vi "Vision Processing.vi"(4 "error in (no error)":errorcluster, 6 "CameraDevRef":T1) -> ()   [LabVIEW 2011]
uses:
  <vilib>/Rock Robotics/WPI/Camera/WPI_CameraDevRef.ctl
  Robot Global Data.vi
  <vilib>/vision/NI_Vision_Development_Module.lvlib
panel:
  in  "Default Shooter Speed Dump":dbl=0.42
  in  "Default Shooter Speed Shoot":dbl=0.705
  in  "Scale":dbl=0.85
  in  "Minimum Power":dbl=0.22
  out "Aspect Ratio":dbl[](array[numeric])
  out "Offset":dbl
  in  "Max Distance for 1 hoop":dbl=8.0
  out "Raw Turret":dbl
  in  "Run Calculations":bool=TRUE
  out "Target X Coord":dbl
  out "Target Distance":dbl
  out "Target Y Coord":dbl
  out "Distance Array":dbl[](array[numeric])
  in  "Dead Band":dbl=0.09
  out "Number of Rectangles Visible":dbl
  out "Y Position Array":dbl[](array[numeric])
  out "X Position Array":dbl[](array[numeric])
  in  "View":bool
  out "Target Info":T2(array[cluster])
  in  "Area Size Limit":i32=444
  in  "Particle Count Limit":i32=8
  in  "Score Limits":T3={"Rect Coverage"=76.0, "Aspect Ratio"=40.0, "X Edge Strength"=40.0, "Y Edge Strength"=60.0}
  in  "Processing":enum32{"Color", "Intensity", "Intensity Open"}(tab)=enum."Intensity"
  in  "Luminance":i32=255
  in  "Saturation":i32=255
  in  "Hue":i32(knob)=65 scale=0.0..255.0
  in  "Margins":cluster{"Hue":i32, "Sat":i32, "Lum":i32}={"Hue"=20, "Sat"=27, "Lum"=30} {"Sat" scale=0.0..40.0; "Lum" scale=0.0..40.0; "Hue" scale=0.0..40.0}
  in  "Range":cluster{"Lower value":sgl, "Upper value":sgl}={"Lower value"=151.52174, "Upper value"=255.0} {"Lower value" scale=0.0..255.0; "Upper value" scale=0.0..255.0}
  in  "Range":cluster{"Lower value":sgl, "Upper value":sgl}={"Lower value"=123.804344, "Upper value"=255.0} {"Lower value" scale=0.0..255.0; "Upper value" scale=0.0..255.0}
  in  "View":bool
  out "Processed Image":T4(plugin-control)
  out "Original Image":T4(plugin-control)
  # "Instructions:\nProcessing the reflective tape that is illuminated by a ring light can be based\non color or light intensity.\nParticles within the image are scored by rectangle coverage, aspect ratio, and\nfor being hollow with a bold edge. A particle is considered a target if all scores\nare above the score limits. Particles can be annotated -- surrounded by\na rectangle and scores drawn to the left .\nTo control the number of particles being scored, use the count limit and the size\nlimit."
  # "(in)"
  # "To debug, Enable using the View button.\nFor color processing, you can click in the image to select the color for processing."
  # "Enable by clicking the View button.\nGreen scores are above the limit, orange are below. Inner/outer rect\nindicates all passed."
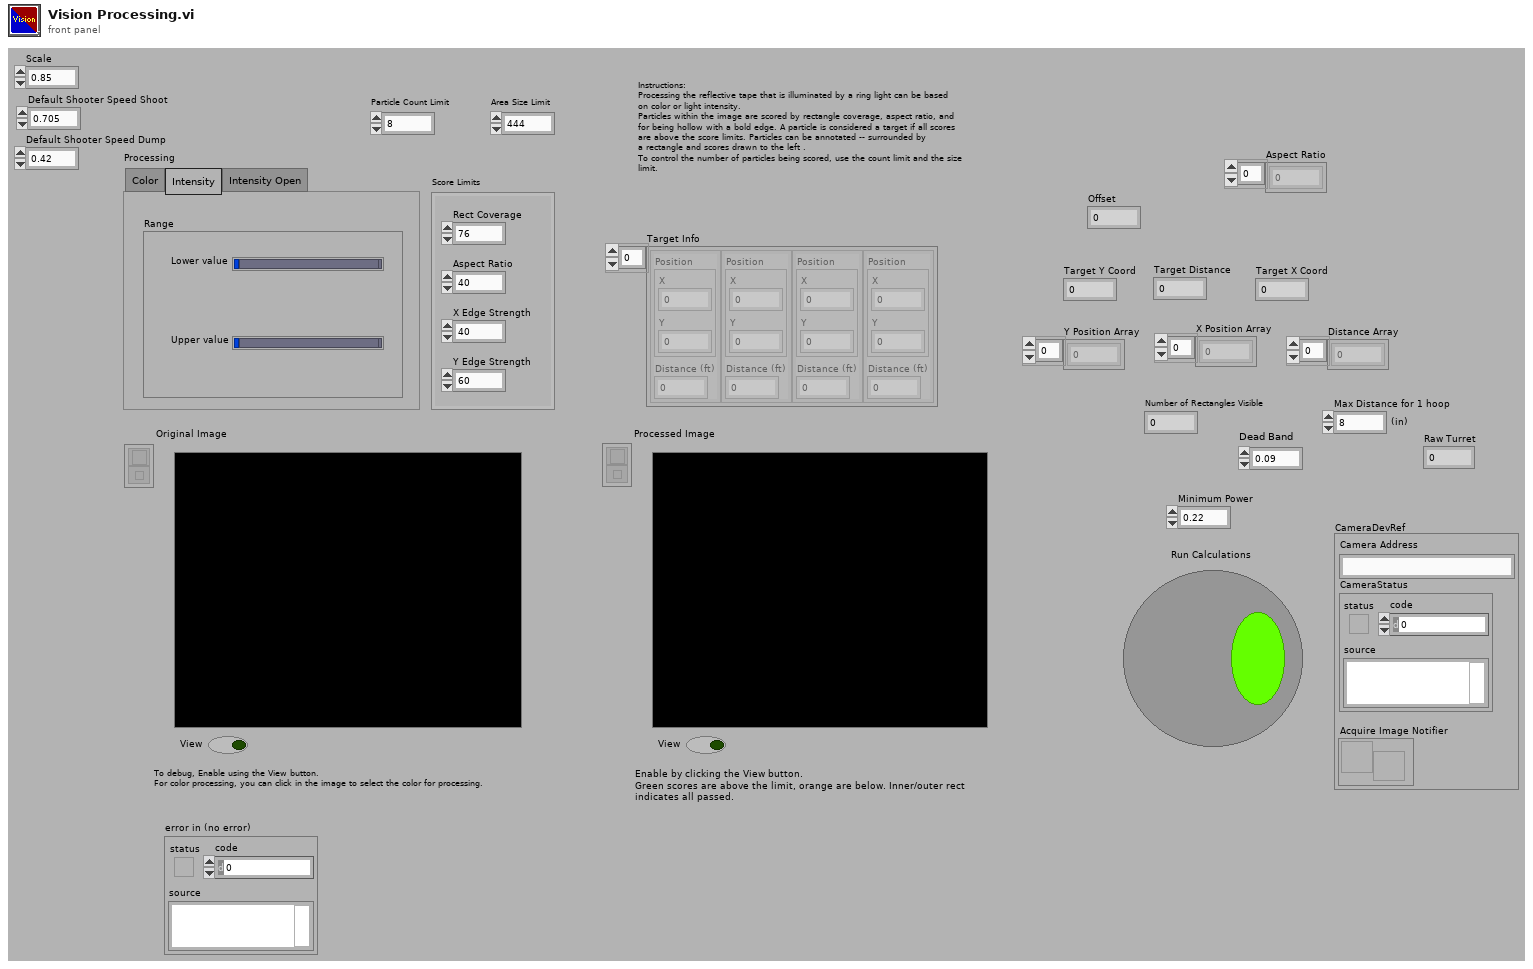
[diagram p1: front panel]
types:
  T1 = typedef "WPI_CameraDevRef.ctl" = cluster{"Camera Address":string, "CameraStatus":errorcluster, "Acquire Image Notifier":refnum<notifier>}
  T2 = cluster{"Position":cluster{"X":dbl, "Y":dbl}, "Distance (ft)":dbl}[]
  T3 = cluster{"Rect Coverage":dbl, "Aspect Ratio":dbl, "X Edge Strength":dbl, "Y Edge Strength":dbl}
  T4 = typedef "IMAQ Image.ctl" = refnum<image>
  T5 = typedef "Image Type" = u32
  T6 = enum32{"AutoM", "Close", "Dilate", "Erode", "Gradient", "Gradient out", "Gradient in", "Hit miss", "Open", "PClose", "POpen", "Thick", "Thin"}
  T7 = typedef "WPI_CameraImageSize.ctl" = enum16{"640x480", "320x240", "160x120"}
  T8 = cluster{"fps":i32, "compression":i32, "Image Size":T7}
  T9 = cluster{cluster{"Left":dbl, "Top":dbl, "Right":dbl, "Bottom":dbl}, dbl[]}[]
  T10 = cluster{"Left":dbl, "Top":dbl, "Right":dbl, "Bottom":dbl}
  T11 = cluster{"Target Center (-1 to 1)":cluster{"X":dbl, "Y":dbl}, "Distance (ft)":dbl}
  T12 = cluster{"Target Center (-1 to 1)":cluster{"X":dbl, "Y":dbl}, "Distance (ft)":dbl}[]
  T13 = typedef "WPI_JoystickDevRef.ctl" = cluster{"Device":T14}
  T14 = typedef "WPI_JoystickDeviceEnum.ctl" = enum16{"USB 1", "USB 2", "USB 3", "USB 4", "Kinect 1", "Kinect 2"}
  T15 = typedef "WPI_JoystickButtonState.ctl" = cluster{"Button 1":bool, "Button 2":bool, "Button 3":bool, "Button 4":bool, "Button 5":bool, "Button 6":bool, "Button 7":bool, "Button 8":bool, "Button 9":bool, "Button 10":bool, "Button 11":bool, "Button 12":bool}
  T16 = cluster{"axis 1 (x)":dbl, "axis 2 (y)":dbl, "axis 3 (throttle)":dbl, "axis 4":dbl, "axis 5":dbl, "axis 6":dbl}
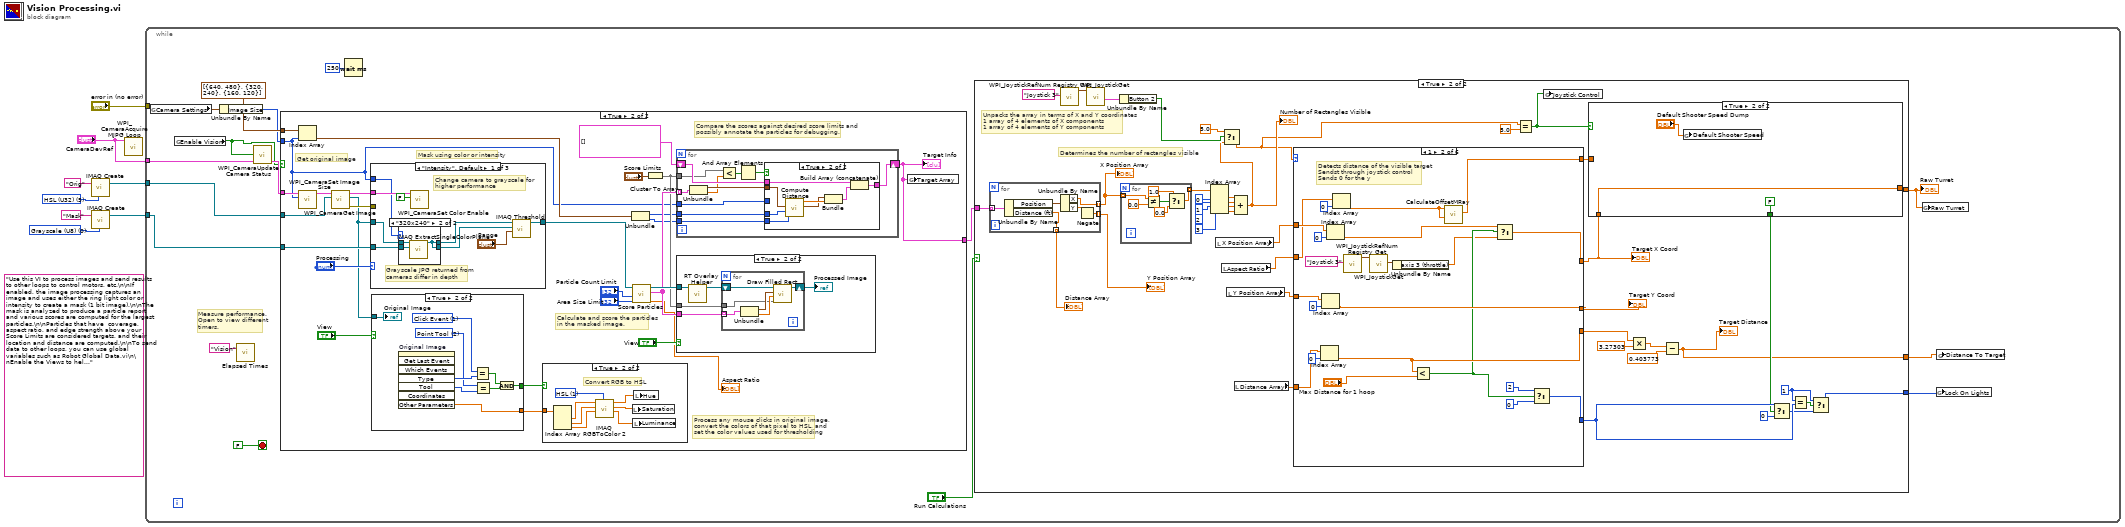
[diagram p0: block diagram]
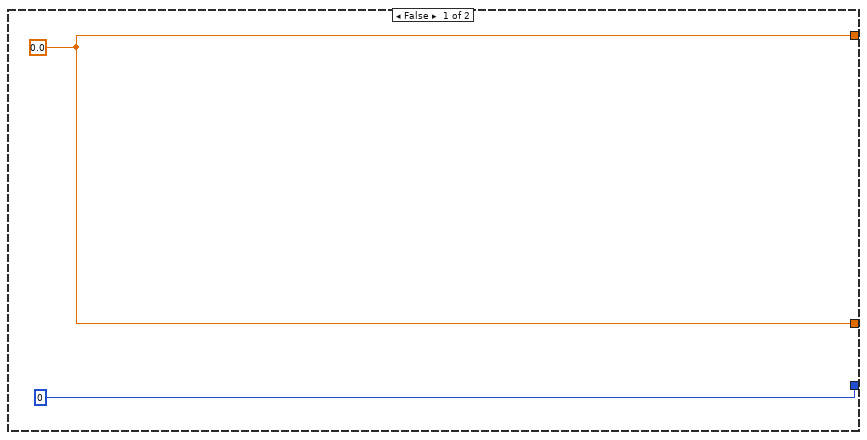
[diagram p2: hidden frame]
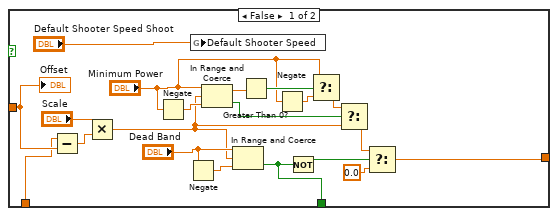
[diagram p3: hidden frame]
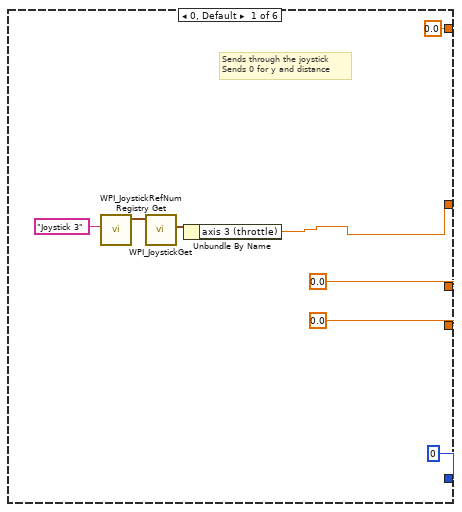
[diagram p4: hidden frame]
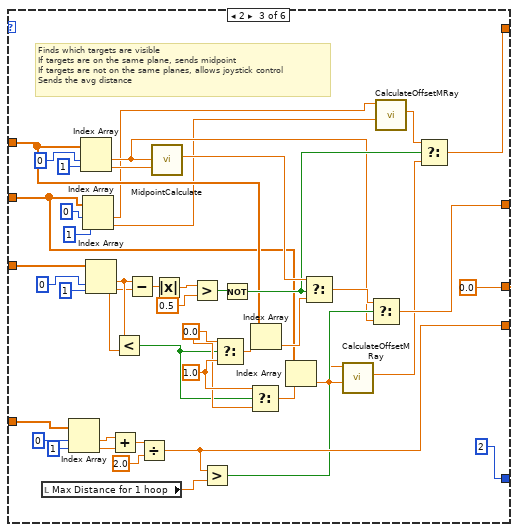
[diagram p5: hidden frame]
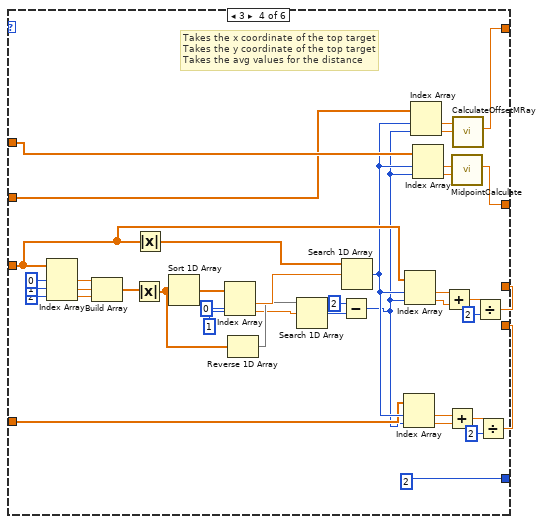
[diagram p6: hidden frame]
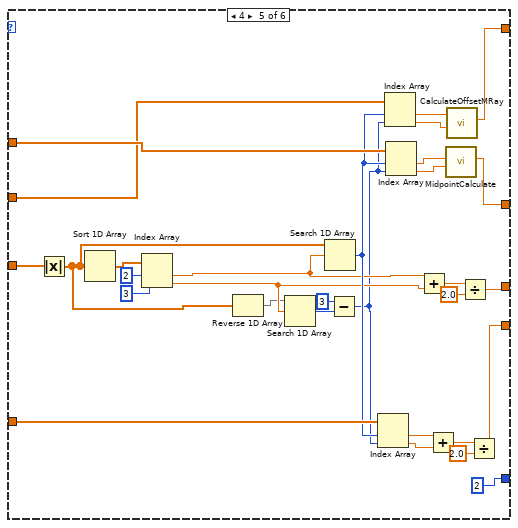
[diagram p7: hidden frame]
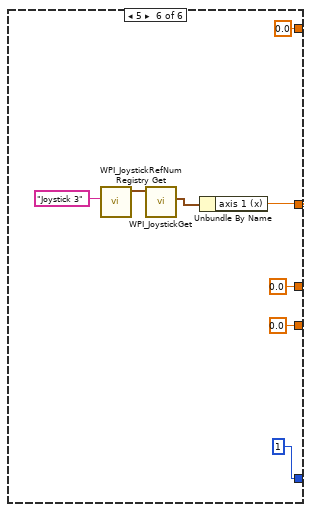
[diagram p8: hidden frame]
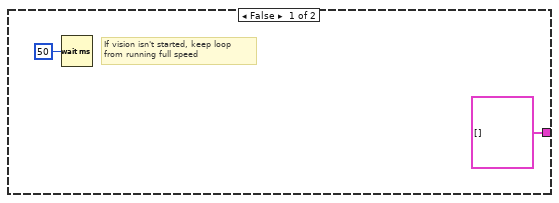
[diagram p9: hidden frame]
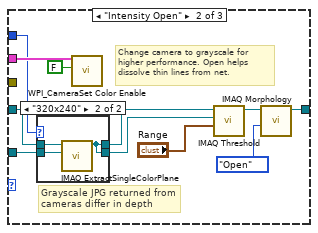
[diagram p12: hidden frame]
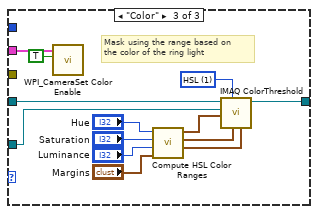
[diagram p14: hidden frame]
diagram:
  w3 = T5 0 items=["Grayscale (U8)", "Grayscale (I16)", "Grayscale (SGL)", "Complex (CSG)", "RGB (U32)", "HSL (U32)", "RGB (U64)", "Grayscale (U16)"] ("Image Type")
  (unwired) "Use this VI to process images and send results to other loops to control motors, etc.\n\nIf enabled, the image processing captures an image and uses either the ring light color or intensity to create a mask (1 bit image).\n\nThe mask is analyzed to produce a particle report and various scores are computed for the largest particles.\n\nParticles that have  coverage, aspect ratio, and edge strength above your Score Limits are considered targets, and their location and distance are computed.\n\nTo send data to other loops, you can use global variables such as Robot Global Data.vi\n\nEnable the Views to help debug color settings. Disable the View to speed up processing."
  w7 = T5 5 items=["Grayscale (U8)", "Grayscale (I16)", "Grayscale (SGL)", "Complex (CSG)", "RGB (U32)", "HSL (U32)", "RGB (U64)", "Grayscale (U16)"] ("Image Type")
  n1 = call "IMAQ Create"("Image Name"="Orig", "Image Type"=w7) -> ("New Image"=w6:T4)  [unwired: 2 in, 2 out]
  n2 = call "IMAQ Create"("Image Name"="Mask", "Image Type"=w3) -> ("New Image"=w1:T4)  [unwired: 2 in, 2 out]
  n3 = call <vilib>:"WPI_CameraAcquire MJPG Loop.vi"("CameraDevRef"="CameraDevRef") -> ()  [unwired: 11 in]
  n4 = while {
    tunnel: w6 -> [w23]
    tunnel: "CameraDevRef" -> [w22]
    tunnel: "error in (no error)" -> [_]
    tunnel: w1 -> [w18]
    stop <- FALSE stop-if-true
    # "Measure performance.\nOpen to view different\ntimers."
    n5 = global read "Robot Global Data.vi" "Camera Settings"() -> (w16:T8)
    n6 = global read "Robot Global Data.vi" "Enable Vision"() -> (w20:bool)
    n7 = Unbundle By Name(w16) -> ("Image Size"=w15:T7)
    n8 = call "Elapsed Times.vi"("Call Name"="Vision") -> ()  [unwired: 2 in, 1 out]
    n9 = call <vilib>:"WPI_CameraUpdate Camera Status.vi"("CameraDevRef In"=w22, "Enable Vision"=w20) -> ("CameraDevRef Out"=w21:T1)  [unwired: 3 in]
    n10 = case shown="True" w20 {
      tunnel: w23 -> [_ w277]
      tunnel: w21 -> [_ w273]
      tunnel: w18 -> [_ w264]
      tunnel: cluster{i32, i32}[] [{640, 480}, {320, 240}, {160, 120}] -> [_ w268]
      tunnel: w15 -> [_ w261]
      tunnel: [T2 [] w262] -> w14
      frame False {
        # "If vision isn't started, keep loop\nfrom running full speed"
        n11 = Wait (ms)(milliseconds to wait=u32 50) -> ()  [unwired: 1 out]
      }
      frame True {
        # "Compare the scores against desired score limits and\npossibly annotate the particles for debugging."
        # "Process any mouse clicks in original image,\nconvert the colors of that pixel to HSL, and\nset the color values used for thresholding"
        # "Calculate and score the particles\nin the masked image."
        # "Mask using color or intensity"
        # "Get original image"
        n12 = call <vilib>:"WPI_CameraSet Image Size.vi"("Image Size"=w261, "CameraDevRef"=w273) -> ("CameraDevRef Out"=w274:T1)  [unwired: 8 in, 1 out]
        n13 = Index Array(array=w268, index=w261) -> (element=w265:cluster{i32, i32})
        n14 = call <vilib>:"WPI_CameraGet Image.vi"("Image"=w277, "CameraDevRef"=w274) -> ("error out"=w275:errorcluster, "Image Out"=w263:T4, "CameraDevRef Out"=w276:T1)  [unwired: 7 in]
        n15 = case shown="\"Intensity\", Default" "Processing" {
          tunnel: w263 -> [w299 w311 w337]
          tunnel: [w302 w316 w336] -> w271
          tunnel: w276 -> [w300 w314 w327]
          tunnel: w275 -> [_ _ _]
          tunnel: w264 -> [w298 w312 w325]
          tunnel: w261 -> [w297 w313 _]
          frame "Intensity", Default {
            # "Grayscale JPG returned from\ncameras differ in depth"
            # "Change camera to grayscale for\nhigher performance"
            n16 = case shown="\"320x240\"" w297 {
              tunnel: w299 -> [w305 w308]
              tunnel: w298 -> [w304 w307]
              tunnel: [w305 w306] -> w296
              tunnel: [w304 w306] -> w295
              frame "640x480", Default {
              }
              frame "320x240" {
                n17 = call "IMAQ ExtractSingleColorPlane"("Image Dst"=w307, "Image Src"=w308) -> ("Image Dst Out"=w306:T4)  [unwired: 8 in, 1 out]
              }
            }
            n18 = call <vilib>:"WPI_CameraSet Color Enable.vi"("Color Enabled"=FALSE, "CameraDevRef"=w300) -> ()  [unwired: 8 in, 2 out]
            n19 = call "IMAQ Threshold"("Range"="Range", "Image Dst"=w295, "Image Src"=w296) -> ("Image Dst Out"=w302:T4)  [unwired: 3 in, 5 out]
          }
          frame "Intensity Open" {
            # "Grayscale JPG returned from\ncameras differ in depth"
            # "Change camera to grayscale for\nhigher performance. Open helps\ndissolve thin lines from net."
            n20 = case shown="\"320x240\"" w313 {
              tunnel: w311 -> [w321 w324]
              tunnel: w312 -> [w320 w323]
              tunnel: [w321 w322] -> w310
              tunnel: [w320 w322] -> w309
              frame "640x480", Default {
              }
              frame "320x240" {
                n21 = call "IMAQ ExtractSingleColorPlane"("Image Dst"=w323, "Image Src"=w324) -> ("Image Dst Out"=w322:T4)  [unwired: 8 in, 1 out]
              }
            }
            n22 = call <vilib>:"WPI_CameraSet Color Enable.vi"("Color Enabled"=FALSE, "CameraDevRef"=w314) -> ()  [unwired: 8 in, 2 out]
            n23 = call "IMAQ Threshold"("Range"="Range", "Image Dst"=w309, "Image Src"=w310) -> ("Image Dst Out"=w317:T4)  [unwired: 3 in, 5 out]
            n24 = call "IMAQ Morphology"("Operation"=T6."Open", "Image Src"=w317) -> ("Image Dst Out"=w316:T4)  [unwired: 8 in, 1 out]
          }
          frame "Color" {
            w335 = u16 1 items=["RGB", "HSL", "HSV", "HSI"] ("Color Mode")
            # "Mask using the range based on\nthe color of the ring light"
            n25 = call <vilib>:"WPI_CameraSet Color Enable.vi"("Color Enabled"=TRUE, "CameraDevRef"=w327) -> ()  [unwired: 8 in, 2 out]
            n26 = call "Compute HSL Color Ranges.vi"("Margins"="Margins", "Luminance"="Luminance", "Saturation"="Saturation", "Hue"="Hue") -> ("Lum Range"=w332:cluster{i32, i32}, "Sat Range"=w333:cluster{i32, i32}, "Hue Range"=w334:cluster{i32, i32})  [unwired: 5 in]
            n27 = call "IMAQ ColorThreshold"("Blue or Luma or Val or Inten Range"=w332, "Green or Sat Range"=w333, "Color Mode"=w335, "Red or Hue Range"=w334, "Image Dst"=w325, "Image Src"=w337) -> ("Image Dst Out"=w336:T4)  [unwired: 4 in, 1 out]
          }
        }
        n28 = case shown="True" "View" {
          tunnel: w263 -> [_ w357]
          tunnel: [_ w352] -> w270
          tunnel: [_ w349] -> w269
          frame False {
          }
          frame True {
            w350 = 2 items=["None", "Selection Tool", "Point Tool", "Line Tool", "Rectangle Tool", "Oval Tool", "Polygon Tool", "ClosedFreehandTool", "Annulus Tool", "Rotated Rectangle Tool", "Zoom Tool", "Pan Tool", "Polyline Tool", "Freehand Tool"] ("Tool")
            w351 = 1 items=["No Event"=0, "Click Event"=1, "Draw Event"=2, "Size Event"=4, "Scroll Event"=5, "Double Click Event"=8] ("Type")
            n29 = invoke on="Original Image" class="ImageControl" method="Get Last Event"() -> ("Type"=w353:i32, "Tool"=w356:i32, "Other Parameters"=w349:sgl[])  [unwired: 8 in, 5 out]
            n30 = Equal?(x=w351, y=w353) -> (x = y?=w354:bool)
            n31 = Equal?(x=w350, y=w356) -> (x = y?=w355:bool)
            n32 = And(x=w354, y=w355) -> (x .and. y?=w352:bool)
            "Original Image" <- w357
          }
        }
        n33 = case shown="True" w270 {
          tunnel: w269 -> [_ w294]
          frame False {
          }
          frame True {
            w293 = u16 1 items=["RGB", "HSL", "HSV", "HSI", "CIE L*a*b*", "CIE XYZ"] ("Color Mode")
            # "Convert RGB to HSL"
            n34 = Index Array(array=w294) -> (element #1=w292:sgl, element #2=w290:sgl, element #3=w288:sgl)  [unwired: 3 in]
            n35 = call "IMAQ RGBToColor 2"("Color Mode"=w293, "Blue value"=w288, "Green value"=w290, "Red value"=w292) -> ("Blue or Luma or Val or Inten or Z or b*value"=w287:dbl, "Green or Sat or Y or a* value"=w289:dbl, "Red or Hue or X or L* value"=w291:dbl)  [unwired: 4 in, 1 out]
            n36 = local write "Saturation"(w289) -> ()
            n37 = local write "Luminance"(w287) -> ()
            n38 = local write "Hue"(w291) -> ()
          }
        }
        n39 = Unbundle(w265) -> (w267:i32, w266:i32)
        n40 = call "Score Particles.vi"("Area Size Limit"="Area Size Limit", "Particle Count Limit"="Particle Count Limit", "Image Refnum in"=w271) -> ("Aspect Ratio"=→"Aspect Ratio":dbl[], "Scored Particle Info"=w282:T9, "Image Refnum out"=w285:T4)  [unwired: 6 in]
        n41 = Cluster To Array(cluster="Score Limits") -> (array=w280:dbl[])
        n42 = for {
          shift-right: [w367] -> w262
          shift-left: T2 [] -> [w368]
          tunnel: w267 -> [w366]
          tunnel: w282 -> [w364] mode=indexing
          tunnel: w280 -> [w359]
          tunnel: w261 -> [w363]
          tunnel: w266 -> [w358]
          n43 = Unbundle(w364) -> (w365:T10, w360:dbl[])
          n44 = Less?(x=w359, y=w360) -> (x < y?=w362:bool[])
          n45 = And Array Elements(Boolean array=w362) -> (logical AND=w361:bool)
          n46 = case shown="True" w361 {
            tunnel: w368 -> [w369 w377]
            tunnel: [w369 w376] -> w367
            tunnel: w365 -> [_ w372]
            tunnel: w366 -> [_ w374]
            tunnel: w363 -> [_ _]
            tunnel: w358 -> [_ w371]
            frame False {
            }
            frame True {
              n47 = call "Compute Distance.vi"("Y Image Resolution"=w371, "X Image Resolution"=w374, "Bounding Box"=w372) -> ("Target Center (-1 to 1)"=w370:cluster{"X":dbl, "Y":dbl}, "Distance (ft)"=w373:dbl)  [unwired: 7 in]
              n48 = Bundle("Target Center (-1 to 1)"=w370, "Distance (ft)"=w373) -> (w375:T11)  [unwired: 1 in]
              n49 = Build Array (concatenate)(w377, w375) -> (w376:T12)
            }
          }
        }
        "Target Info" <- w262
        n50 = case shown="True" "View" {
          tunnel: w285 -> [_ w339]
          tunnel: w282 -> [_ w341]
          tunnel: w280 -> [_ w340]
          frame False {
          }
          frame True {
            n51 = call "RT Overlay Helper.vi"("Refnum in"=w339) -> ("Refnum out"=w342:T4)  [unwired: 10 in]
            n52 = for {
              shift-right: [w347] -> w338
              shift-left: w342 -> [w348]
              tunnel: w341 -> [w344] mode=indexing
              tunnel: w340 -> [w343]
              n53 = Unbundle(w344) -> (w345:T10, w346:dbl[])
              n54 = call "Draw Filled Rect.vi"("Limits"=w343, "Scores"=w346, "Bounding Box"=w345, "image in"=w348) -> ("image out"=w347:T4)  [unwired: 7 in]
            }
            "Processed Image" <- w338
          }
        }
        n55 = global write "Robot Global Data.vi" "Target Array"(w262) -> ()
      }
    }
    n56 = Wait (ms)(milliseconds to wait=u32 250) -> ()  [unwired: 1 out]
    n57 = case shown="True" "Run Calculations" {
      tunnel: w14 -> [_ w51]
      tunnel: [w25 w36] -> w11
      tunnel: [0 ("f") w44] -> w10
      tunnel: [w25 w28] -> w9
      frame False {
        w25 = 0.0 ("f")
      }
      frame True {
        w45 = 1 ("y")
        # "Determines the number of rectangles visible"
        # "Unpacks the array in terms of X and Y coordinates\n1 array of 4 elements of X components\n1 array of 4 elements of Y components"
        n58 = for {
          tunnel: [w255] -> w52 mode=indexing
          tunnel: [w256] -> w62 mode=indexing
          tunnel: w51 -> [w253] mode=indexing
          tunnel: [w252] -> w64 mode=indexing
          n59 = Unbundle By Name(w253) -> ("Position"=w257:cluster{"X":dbl, "Y":dbl}, "Distance (ft)"=w252:dbl)
          n60 = Unbundle By Name(w257) -> ("X"=w256:dbl, "Y"=w254:dbl)
          n61 = Negate(x=w254) -> (-x=w255:dbl)
        }
        "X Position Array" <- w62
        "Y Position Array" <- w52
        "Distance Array" <- w64
        n62 = call <vilib>:"WPI_JoystickRefNum Registry Get.vi"("refnum name"="Joystick 3") -> ("JoystickDevRef"=w50:T13)  [unwired: 9 in, 1 out]
        n63 = call <vilib>:"WPI_JoystickGet.vi"("JoystickDevRef"=w50) -> ("Buttons"=w48:T15)  [unwired: 4 in, 2 out]
        n64 = Unbundle By Name(w48) -> ("Button 2"=w47:bool)
        n65 = for {
          tunnel: w62 -> [w96] mode=indexing
          tunnel: [w92] -> w61 mode=indexing
          n66 = Not Equal?(x=w96, y=0.0) -> (x != y?=w95:bool)
          n67 = Select(t=1.0, s=w95, f=0.0) -> (s? t:f=w92:dbl)
        }
        n68 = Index Array(array=w61, index #1=0 ("index"), index #2=1 ("index"), index #3=2 ("index"), index #4=3 ("index")) -> (element #1=w59:dbl, element #2=w60:dbl, element #3=w58:dbl, element #4=w57:dbl)
        n69 = local read "X Position Array"() -> (w63:dbl[])
        n70 = local read "Aspect Ratio"() -> (w39:dbl[])
        n71 = local read "Y Position Array"() -> (w66:dbl[])
        n72 = Compound Arithmetic op=ADD(w59, w60, w58, w57) -> (w40:dbl)
        "Number of Rectangles Visible" <- w40
        n73 = Select(t=5.0, s=w47, f=w40) -> (s? t:f=w33:dbl)
        n74 = local read "Distance Array"() -> (w67:dbl[])
        n75 = case shown="1" w33 {
          tunnel: w63 -> [_ w125 w140 w199 w239 _]
          tunnel: [w99 w119 w149 w180 w235 w245] -> w37
          tunnel: [0.0 ("X") w116 0.0 ("X") w200 w234 0.0 ("X")] -> w65
          tunnel: [0.0 ("X") w121 w152 w190 w229 0.0 ("X")] -> w29
          tunnel: w66 -> [_ w117 w171 w195 w243 _]
          tunnel: w67 -> [_ w128 w159 w182 w238 _]
          tunnel: [0 w112 2 2 2 1] -> w43
          tunnel: [0.0 ("Offset") w109 w137 w187 w225 0.0 ("Offset")] -> w38
          tunnel: w39 -> [_ w108 w132 w183 w221 _]
          frame 0, Default {
            # "Sends through the joystick\nSends 0 for y and distance"
            n76 = call <vilib>:"WPI_JoystickRefNum Registry Get.vi"("refnum name"="Joystick 3") -> ("JoystickDevRef"=w103:T13)  [unwired: 9 in, 1 out]
            n77 = call <vilib>:"WPI_JoystickGet.vi"("JoystickDevRef"=w103) -> ("Axes"=w101:T16)  [unwired: 4 in, 2 out]
            n78 = Unbundle By Name(w101) -> ("axis 3 (throttle)"=w99:dbl)
          }
          frame 1 {
            # "Detects distance of the visible target\nSendst through joystick control\nSends 0 for the y"
            n79 = Index Array(array=w128, index=0) -> (element=w121:dbl)
            n80 = Index Array(array=w117, index=0) -> (element=w116:dbl)
            n81 = Index Array(array=w125, index=0) -> (element=w110:dbl)
            n82 = Index Array(array=w108, index=0) -> (element=w106:dbl)
            n83 = call <vilib>:"WPI_JoystickRefNum Registry Get.vi"("refnum name"="Joystick 3") -> ("JoystickDevRef"=w124:T13)  [unwired: 9 in, 1 out]
            n84 = call <vilib>:"WPI_JoystickGet.vi"("JoystickDevRef"=w124) -> ("Axes"=w122:T16)  [unwired: 4 in, 2 out]
            n85 = Unbundle By Name(w122) -> ("axis 3 (throttle)"=w111:dbl)
            n86 = Less?(x=w121, y="Max Distance for 1 hoop") -> (x < y?=w114:bool)
            n87 = call "CalculateOffsetMRay.vi"("AR2"=w106, "AR1"=w106) -> ("Offset"=w109:dbl)  [unwired: 9 in]
            n88 = Select(t=w110, s=w114, f=w111) -> (s? t:f=w119:dbl)
            n89 = Select(t=2, s=w114, f=0) -> (s? t:f=w112:i32)
          }
          frame 2 {
            w143 = 1.0 ("f")
            w142 = 0.0 ("t")
            # "Finds which targets are visible\nIf targets are on the same plane, sends midpoint\nIf targets are not on the same planes, allows joystick control\nSends the avg distance"
            n90 = local read "Max Distance for 1 hoop"() -> (w151:dbl)
            n91 = Index Array(array=w159, index #1=0 ("index"), index #2=1 ("index")) -> (element #1=w158:dbl, element #2=w157:dbl)
            n92 = Index Array(array=w140, index #1=0 ("index"), index #2=1 ("index")) -> (element #1=w146:dbl, element #2=w145:dbl)
            n93 = Index Array(array=w132, index #1=0 ("index"), index #2=1 ("index")) -> (element #1=w134:dbl, element #2=w133:dbl)
            n94 = Index Array(array=w171, index #1=0 ("index"), index #2=1 ("index")) -> (element #1=w131:dbl, element #2=w130:dbl)
            n95 = Add(x=w158, y=w157) -> (x+y=w162:dbl)
            n96 = Less?(x=w131, y=w130) -> (x < y?=w129:bool)
            n97 = Subtract(x=w131, y=w130) -> (x-y=w168:dbl)
            n98 = Divide(x=w162, y=2.0) -> (x/y=w152:dbl)
            n99 = call "MidpointCalculate.vi"("X2"=w145, "X1"=w146) -> ("Midpoint"=w164:dbl)  [unwired: 9 in]
            n100 = Absolute Value(x=w168) -> (abs(x)=w167:dbl)
            n101 = Greater?(x=w167, y=0.5) -> (0:w165:bool)
            n102 = Greater?(x=w152, y=w151) -> (0:w150:bool)
            n103 = Select(t=w142, s=w129, f=w143) -> (s? t:f=w155:dbl)
            n104 = Not(x=w165) -> (.not. x?=w147:bool)
            n105 = Select(t=w143, s=w129, f=w142) -> (s? t:f=w141:dbl)
            n106 = Index Array(array=w140, index=w155) -> (element=w154:dbl)
            n107 = Index Array(array=w132, index=w141) -> (element=w139:dbl)
            n108 = Select(t=w164, s=w147, f=w154) -> (s? t:f=w148:dbl)
            n109 = call "CalculateOffsetMRay.vi"("AR2"=w139, "AR1"=w139) -> ("Offset"=w138:dbl)  [unwired: 9 in]
            n110 = Select(t=w148, s=w150, f=w146) -> (s? t:f=w149:dbl)
            n111 = call "CalculateOffsetMRay.vi"("AR2"=w133, "AR1"=w134) -> ("Offset"=w144:dbl)  [unwired: 9 in]
            n112 = Select(t=w144, s=w147, f=w138) -> (s? t:f=w137:dbl)
          }
          frame 3 {
            # "Takes the x coordinate of the top target\nTakes the y coordinate of the top target\nTakes the avg values for the distance"
            n113 = Index Array(array=w195, index #1=0 ("index"), index #2=1 ("index"), index #3=2 ("index")) -> (element #1=w210:dbl, element #2=w209:dbl, element #3=w208:dbl)
            n114 = Build Array(w210, w209, w208) -> (w207:dbl[])
            n115 = Absolute Value(x=w207) -> (abs(x)=w178:dbl[])
            n116 = Absolute Value(x=w195) -> (abs(x)=w198:dbl[])
            n117 = Sort 1D Array(array=w178) -> (sorted array=w206:dbl[])
            n118 = Index Array(array=w206, index #1=0 ("index"), index #2=1 ("index")) -> (element #1=w203:dbl, element #2=w176:dbl)
            n119 = Reverse 1D Array(array=w178) -> (reversed array=w177:dbl[])
            n120 = Search 1D Array(1D array=w177, element=w176) -> (index of element=w179:i32)  [unwired: 1 in]
            n121 = Subtract(x=2, y=w179) -> (x-y=w174:i32)
            n122 = Search 1D Array(1D array=w198, element=w203) -> (index of element=w186:i32)  [unwired: 1 in]
            n123 = Index Array(array=w182, index #1=w186, index #2=w174) -> (element #1=w192:dbl, element #2=w191:dbl)
            n124 = Index Array(array=w195, index #1=w186, index #2=w174) -> (element #1=w197:dbl, element #2=w196:dbl)
            n125 = Index Array(array=w183, index #1=w186, index #2=w174) -> (element #1=w185:dbl, element #2=w184:dbl)
            n126 = Index Array(array=w199, index #1=w186, index #2=w174) -> (element #1=w181:dbl, element #2=w188:dbl)
            n127 = Add(x=w197, y=w196) -> (x+y=w202:dbl)
            n128 = Add(x=w192, y=w191) -> (x+y=w193:dbl)
            n129 = call "MidpointCalculate.vi"("X2"=w188, "X1"=w181) -> ("Midpoint"=w180:dbl)  [unwired: 9 in]
            n130 = call "CalculateOffsetMRay.vi"("AR2"=w184, "AR1"=w185) -> ("Offset"=w187:dbl)  [unwired: 9 in]
            n131 = Divide(x=w202, y=2) -> (x/y=w200:dbl)
            n132 = Divide(x=w193, y=2) -> (x/y=w190:dbl)
          }
          frame 4 {
            n133 = Absolute Value(x=w243) -> (abs(x)=w217:dbl[])
            n134 = Sort 1D Array(array=w217) -> (sorted array=w242:dbl[])
            n135 = Index Array(array=w242, index #1=2 ("index"), index #2=3 ("index")) -> (element #1=w220:dbl, element #2=w219:dbl)
            n136 = Reverse 1D Array(array=w217) -> (reversed array=w218:dbl[])
            n137 = Search 1D Array(1D array=w218, element=w219) -> (index of element=w216:i32)  [unwired: 1 in]
            n138 = Search 1D Array(1D array=w217, element=w220) -> (index of element=w224:i32)  [unwired: 1 in]
            n139 = Subtract(x=3, y=w216) -> (x-y=w215:i32)
            n140 = Index Array(array=w238, index #1=w224, index #2=w215) -> (element #1=w231:dbl, element #2=w230:dbl)
            n141 = Index Array(array=w221, index #1=w224, index #2=w215) -> (element #1=w222:dbl, element #2=w223:dbl)
            n142 = Index Array(array=w239, index #1=w224, index #2=w215) -> (element #1=w227:dbl, element #2=w226:dbl)
            n143 = Add(x=w220, y=w219) -> (x+y=w237:dbl)
            n144 = Add(x=w231, y=w230) -> (x+y=w232:dbl)
            n145 = call "MidpointCalculate.vi"("X2"=w226, "X1"=w227) -> ("Midpoint"=w235:dbl)  [unwired: 9 in]
            n146 = call "CalculateOffsetMRay.vi"("AR2"=w223, "AR1"=w222) -> ("Offset"=w225:dbl)  [unwired: 9 in]
            n147 = Divide(x=w237, y=2.0) -> (x/y=w234:dbl)
            n148 = Divide(x=w232, y=2.0) -> (x/y=w229:dbl)
          }
          frame 5 {
            n149 = call <vilib>:"WPI_JoystickRefNum Registry Get.vi"("refnum name"="Joystick 3") -> ("JoystickDevRef"=w249:T13)  [unwired: 9 in, 1 out]
            n150 = call <vilib>:"WPI_JoystickGet.vi"("JoystickDevRef"=w249) -> ("Axes"=w247:T16)  [unwired: 4 in, 2 out]
            n151 = Unbundle By Name(w247) -> ("axis 1 (x)"=w245:dbl)
          }
        }
        "Target Y Coord" <- w65
        "Target X Coord" <- w37
        n152 = Equal?(x=w33, y=5.0) -> (x = y?=w27:bool)
        n153 = global write "Robot Global Data.vi" "Joystick Control"(w27) -> ()
        n154 = case shown="True" w27 {
          tunnel: w38 -> [w87 _]
          tunnel: w37 -> [w86 w91]
          tunnel: [w69 w91] -> w36
          tunnel: [w72 FALSE] -> w35
          frame False {
            n155 = Subtract(x=w86, y=w87) -> (x-y=w84:dbl)
            n156 = Multiply(x="Scale", y=w84) -> (x*y=w75:dbl)
            n157 = Negate(x="Minimum Power") -> (-x=w82:dbl)
            n158 = Negate(x="Dead Band") -> (-x=w88:dbl)
            n159 = global write "Robot Global Data.vi" "Default Shooter Speed"("Default Shooter Speed Shoot") -> ()
            n160 = In Range and Coerce(upper limit="Minimum Power", x=w75, lower limit=w82) -> (coerced(x)=w78:dbl, In Range?=w79:bool)
            n161 = In Range and Coerce(upper limit="Dead Band", x=w75, lower limit=w88) -> (In Range?=w72:bool)  [unwired: 1 out]
            n162 = Greater Than 0?(x=w78) -> (x > 0?=w77:bool)
            n163 = Negate(x="Minimum Power") -> (-x=w74:dbl)
            n164 = Not(x=w72) -> (.not. x?=w73:bool)
            n165 = Select(t="Minimum Power", s=w77, f=w74) -> (s? t:f=w76:dbl)
            n166 = Select(t=w76, s=w79, f=w75) -> (s? t:f=w80:dbl)
            n167 = Select(t=w80, s=w73, f=0.0) -> (s? t:f=w69:dbl)
            "Offset" <- w87
          }
          frame True {
            n168 = global write "Robot Global Data.vi" "Default Shooter Speed"("Default Shooter Speed Dump") -> ()
          }
        }
        n169 = Multiply(x=w29, y=3.27303) -> (x*y=w32:dbl)
        n170 = Subtract(x=w32, y=0.403773) -> (x-y=w28:dbl)
        "Target Distance" <- w28
        n171 = Select(t=w43, s=w35, f=0) -> (s? t:f=w41:i32)
        n172 = Equal?(x=w45, y=w43) -> (x = y?=w46:bool)
        n173 = Select(t=w45, s=w46, f=w41) -> (s? t:f=w44:i32)
      }
    }
    "Raw Turret" <- w11
    n174 = global write "Robot Global Data.vi" "Raw Turret"(w11) -> ()
    n175 = global write "Robot Global Data.vi" "Lock On Lights"(w10) -> ()
    n176 = global write "Robot Global Data.vi" "Distance To Target"(w9) -> ()
  }
